vi "LayerBinString.vi"(10 "BinStringIn":string, 11 "Layer":u16) -> (3 "BinStringOut":string)   [LabVIEW 2012]
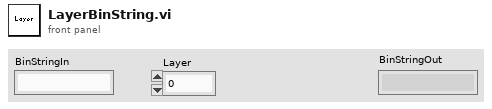
[diagram p1: front panel]
types:
  T1 = enum16{"big-endian, network order", "native, host order", "little-endian"}
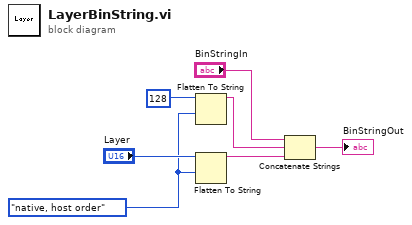
[diagram p0: block diagram]
diagram:
  w2 = T1."native, host order" ("byte order (0:big-endian, network order)")
  n1 = Flatten To String(anything=u16 128 ("Layer"), byte order (0:big-endian, network order)=w2) -> (data string=w4:string)  [unwired: 2 in, 2 out]
  n2 = Flatten To String(anything="Layer", byte order (0:big-endian, network order)=w2) -> (data string=w3:string)  [unwired: 2 in, 2 out]
  n3 = Concatenate Strings("BinStringIn", w4, w3) -> (→"BinStringOut":string)
